vi "read_piecewise_function_file (SubVI).vi"(11 "Path":path) -> (2 "arctan":dbl[][](array[numeric]), 3 "sigmoid":dbl[][](array[numeric]))   [LabVIEW 2020]
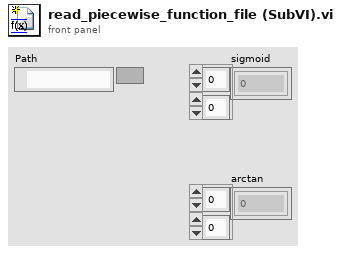
[diagram p1: front panel]
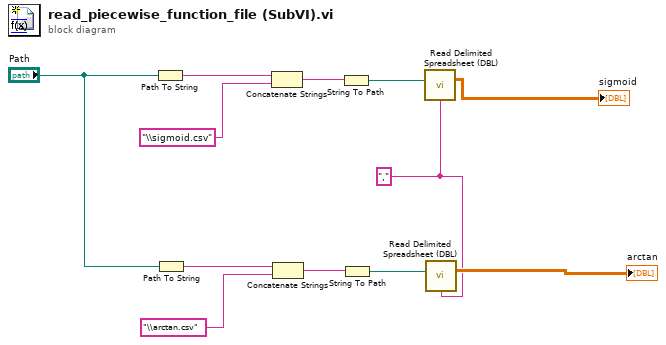
[diagram p0: block diagram]
diagram:
  w10 = ","
  n1 = Path To String(path="Path") -> (string=w1:string)
  n2 = Path To String(path="Path") -> (string=w5:string)
  n3 = Concatenate Strings(w1, "\\sigmoid.csv") -> (w3:string)
  n4 = Concatenate Strings(w5, "\\arctan.csv") -> (w7:string)
  n5 = String To Path(string=w3) -> (path=w4:path)
  n6 = String To Path(string=w7) -> (path=w8:path)
  n7 = call <vilib>:"Read Delimited Spreadsheet (DBL).vi"("file path (dialog if empty)"=w4, "delimiter (\\t)"=w10) -> ("all rows"=→"sigmoid":dbl[][])  [unwired: 8 in, 5 out]
  n8 = call <vilib>:"Read Delimited Spreadsheet (DBL).vi"("file path (dialog if empty)"=w8, "delimiter (\\t)"=w10) -> ("all rows"=→"arctan":dbl[][])  [unwired: 8 in, 5 out]
